vi "Assemble DC Rectifier Setting Changes for PLC.vi"(6 "Num Steps":i32, 7 "Rect Number":i32=1, 8 "error In":errorcluster, 10 "message queue in":T1, 11 "MulticolumnListbox in":refnum<vi>) -> (0 "Right Anode Mins":dbl, 1 "Left Anode Mins":dbl, 2 "Right AmpMin":dbl, 3 "Left AmpMin":dbl, 4 "error out":errorcluster)   [LabVIEW 2019]
uses:
  <vilib>/NI/AMC/Message Queue.ctl
  <vilib>/NI/AMC/Message.ctl
  <vilib>/NI/Tools/Keyed Array/KeyedArray.ctl
  <vilib>/NI/Current Value Table/Type Defs/Single Tag.ctl
  <vilib>/NI/Current Value Table/Type Defs/Data Types.ctl
  <vilib>/NI/AMC/Create Single Message.vi
  <vilib>/NI/AMC/Update Message Routing Info.vi
  <vilib>/NI/AMC/Send Message.vi
  <vilib>/NI/AMC/AMC.lvlib
  <vilib>/NI/Current Value Table/Current Value Table.lvlib
  <vilib>/NI/Tools/Keyed Array/Tools_KeyedArray.lvlib
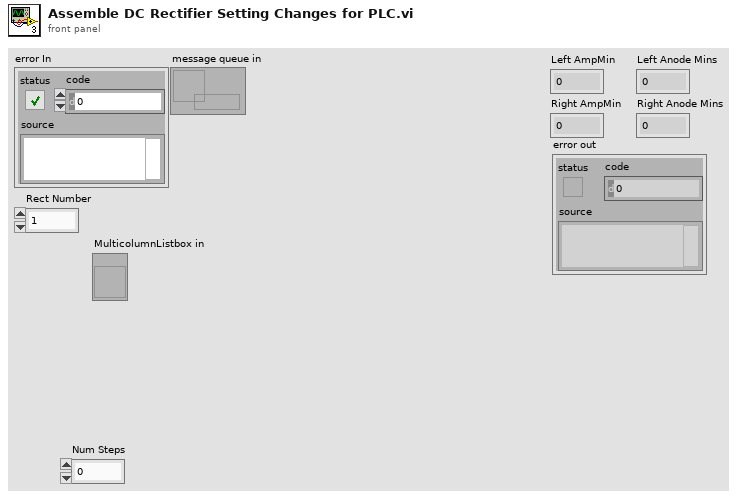
[diagram p1: front panel]
types:
  T1 = typedef "AMC.lvlib/Message Queue.ctl" = refnum<queue>
  T2 = typedef "Current Value Table.lvlib/Data Types.ctl" = enum16{"Double", "Single", "I64", "I32", "I16", "I8", "U64", "U32", "U16", "U8", "String", "Boolean", "Array of U8", "Array of U16", "Array of U32", "Array of U64", "Array of I64", "Array of I32", "Array of I16", "Array of I8", "Array of Double", "Array of Single", "Array of Boolean", "Array of String"}
  T3 = typedef "Current Value Table.lvlib/Single Tag.ctl" = cluster{"Data Type":T2, "Name":string, "Value":string, "Description":string}
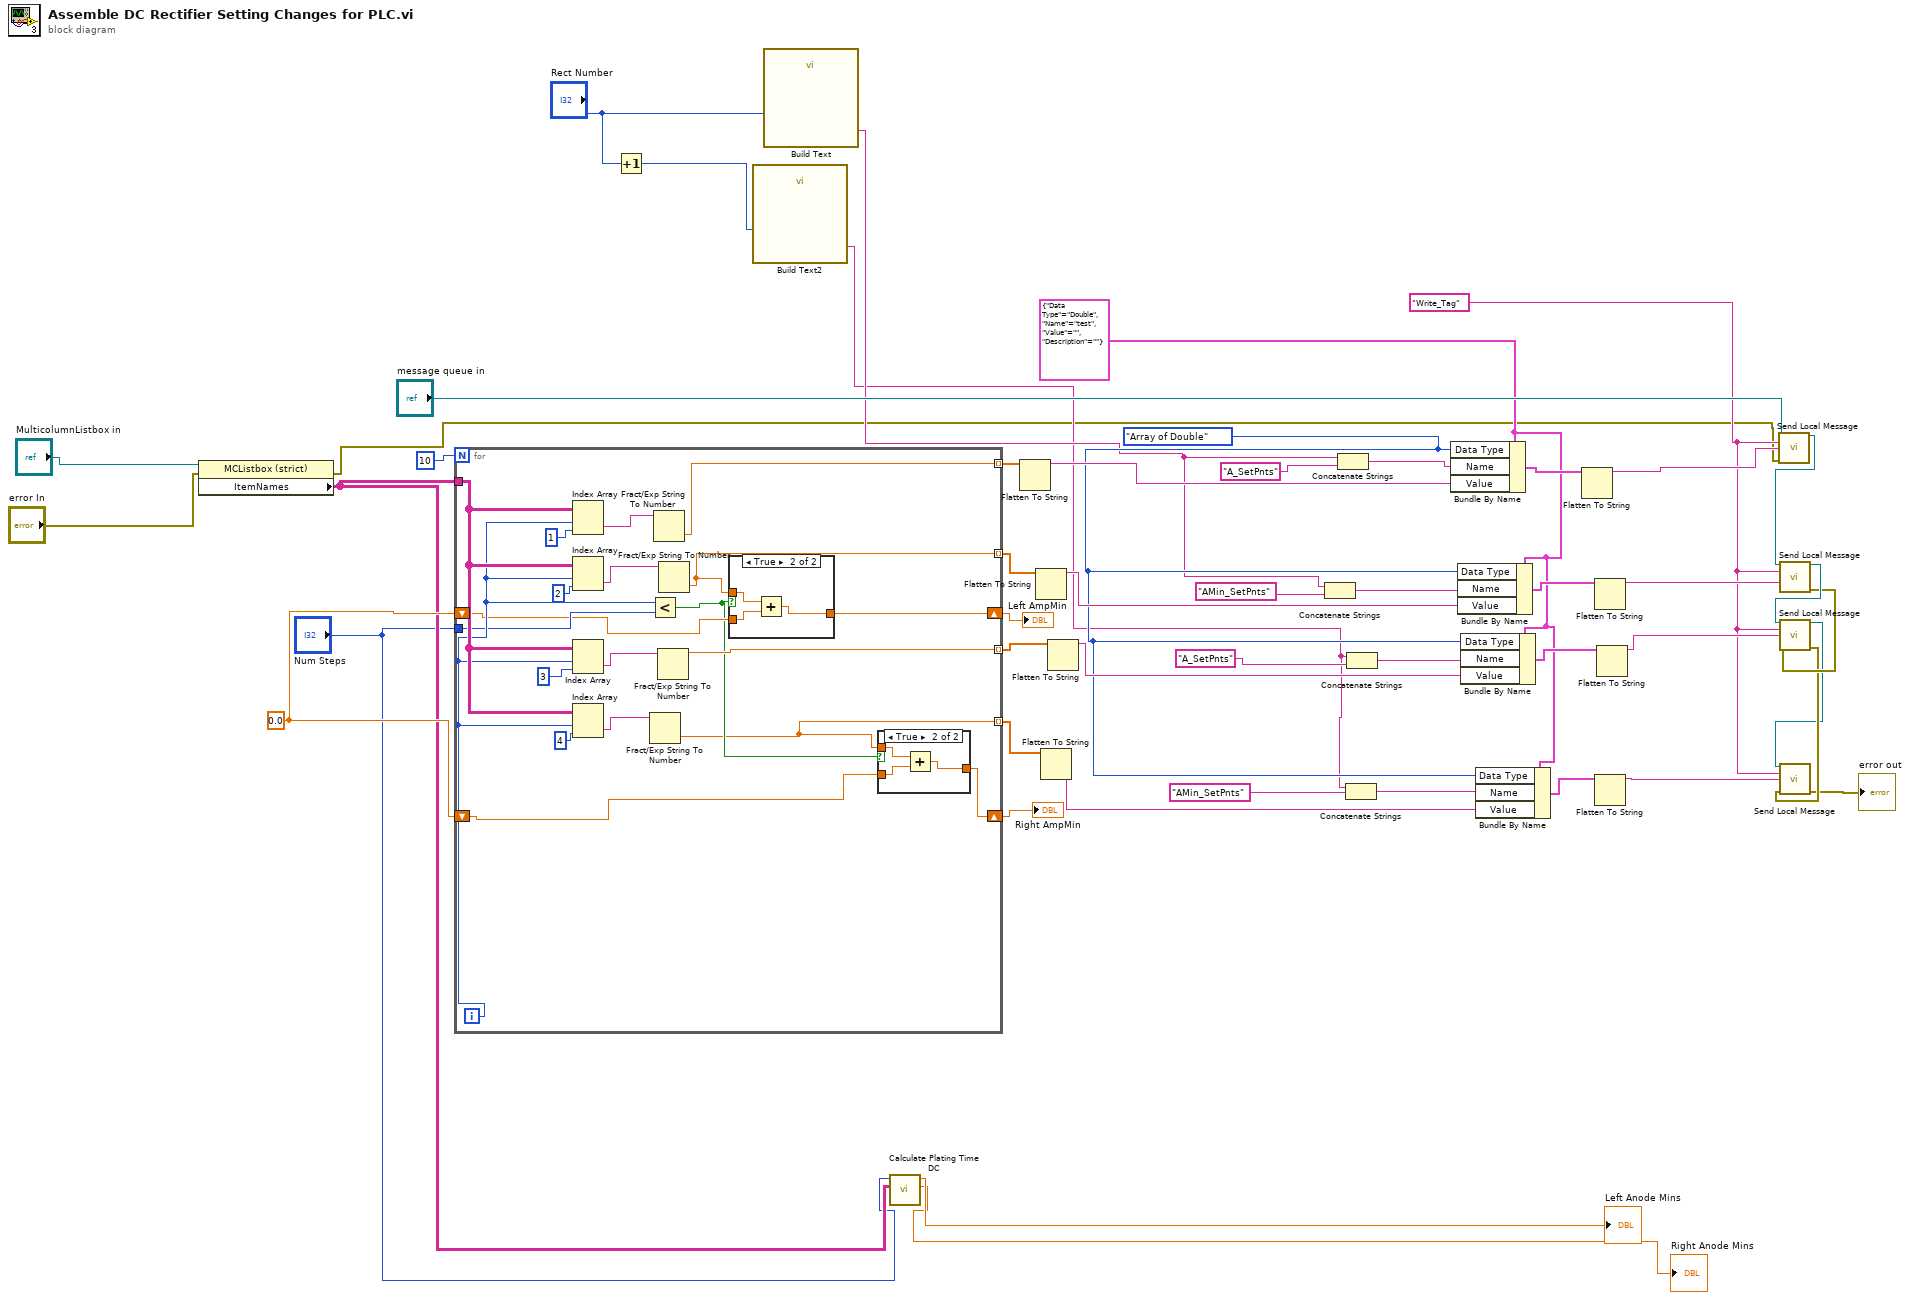
[diagram p0: block diagram]
diagram:
  w13 = 0.0
  w27 = Data_Types."Array of Double" ("Data Type")
  w28 = T3 {"Data Type"=enum."Double", "Name"="test", "Value"="", "Description"=""} ("Tag")
  w26 = "Write_Tag" ("message name")
  n1 = property class="MCListbox (strict)"(reference="MulticolumnListbox in", error in="error In") -> (error out=w12:errorcluster, "ItemNames"=w4:string[][])  [unwired: 1 out]
  n2 = for {
    N: 10 -> [_]
    tunnel: w4 -> [w64]
    tunnel: [w60] -> w46 mode=indexing
    tunnel: [w56] -> w41 mode=indexing
    tunnel: [w59] -> w37 mode=indexing
    tunnel: [w52] -> w32 mode=indexing
    tunnel: "Num Steps" -> [w57]
    shift-right: [w54] -> w10
    shift-left: w13 -> [w55]
    shift-right: [w50] -> w9
    shift-left: w13 -> [w51]
    i -> [w58]
    n3 = Index Array(array=w64, index (row)=w58, index (col)=1 ("disabled index (col)")) -> (element=w68:string)
    n4 = Index Array(array=w64, index (row)=w58, index (col)=2 ("disabled index (col)")) -> (element=w63:string)
    n5 = Index Array(array=w64, index (row)=w58, index (col)=3 ("disabled index (col)")) -> (element=w62:string)
    n6 = Index Array(array=w64, index (row)=w58, index (col)=4 ("disabled index (col)")) -> (element=w61:string)
    n7 = Less?(x=w58, y=w57) -> (x < y?=w53:bool)
    n8 = Fract/Exp String To Number(string=w61) -> (number=w52:dbl)  [unwired: 3 in, 1 out]
    n9 = Fract/Exp String To Number(string=w68) -> (number=w60:dbl)  [unwired: 3 in, 1 out]
    n10 = Fract/Exp String To Number(string=w62) -> (number=w59:dbl)  [unwired: 3 in, 1 out]
    n11 = Fract/Exp String To Number(string=w63) -> (number=w56:dbl)  [unwired: 3 in, 1 out]
    n12 = case shown="True" w53 {
      tunnel: w56 -> [_ w77]
      tunnel: w55 -> [w74 w76]
      tunnel: [w74 w75] -> w54
      frame False {
      }
      frame True {
        n13 = Add(x=w77, y=w76) -> (x+y=w75:dbl)
      }
    }
    n14 = case shown="True" w53 {
      tunnel: w52 -> [_ w73]
      tunnel: w51 -> [w70 w72]
      tunnel: [w70 w71] -> w50
      frame False {
      }
      frame True {
        n15 = Add(x=w73, y=w72) -> (x+y=w71:dbl)
      }
    }
  }
  "Left AmpMin" <- w10
  "Right AmpMin" <- w9
  n16 = Increment(x="Rect Number") -> (x+1=w24:i32)
  n17 = call "Build Text2"("Rect1"=w24) -> ("Result"=w15:string)  [unwired: 13 in, 1 out]
  n18 = call "Build Text"("Rect1"="Rect Number") -> ("Result"=w19:string)  [unwired: 13 in, 1 out]
  n19 = call "Calculate Plating Time DC.vi"("ItemNames"=w4, "Num Steps"="Num Steps") -> ("Right Anode Time"=→"Right Anode Mins":dbl, "Left Anode Time"=→"Left Anode Mins":dbl)  [unwired: 8 in]
  n20 = Flatten To String(anything=w46) -> (data string=w44:string)  [unwired: 3 in, 2 out]
  n21 = Flatten To String(anything=w41) -> (data string=w40:string)  [unwired: 3 in, 2 out]
  n22 = Flatten To String(anything=w32) -> (data string=w31:string)  [unwired: 3 in, 2 out]
  n23 = Flatten To String(anything=w37) -> (data string=w36:string)  [unwired: 3 in, 2 out]
  n24 = Concatenate Strings(w19, "AMin_SetPnts" ("Name")) -> (w21:string)
  n25 = Concatenate Strings(w19, "A_SetPnts" ("Name")) -> (w23:string)
  n26 = Concatenate Strings(w15, "AMin_SetPnts" ("Name")) -> (w16:string)
  n27 = Concatenate Strings(w15, "A_SetPnts" ("Name")) -> (w17:string)
  n28 = Bundle By Name(cluster=w28, "Data Type"=w27, "Name"=w23, "Value"=w44) -> (w43:T3)
  n29 = Bundle By Name(cluster=w28, "Data Type"=w27, "Name"=w21, "Value"=w40) -> (w39:T3)
  n30 = Bundle By Name(cluster=w28, "Data Type"=w27, "Name"=w17, "Value"=w36) -> (w35:T3)
  n31 = Bundle By Name(cluster=w28, "Data Type"=w27, "Name"=w16, "Value"=w31) -> (w30:T3)
  n32 = Flatten To String(anything=w43) -> (data string=w42:string)  [unwired: 3 in, 2 out]
  n33 = Flatten To String(anything=w39) -> (data string=w38:string)  [unwired: 3 in, 2 out]
  n34 = Flatten To String(anything=w30) -> (data string=w29:string)  [unwired: 3 in, 2 out]
  n35 = Flatten To String(anything=w35) -> (data string=w33:string)  [unwired: 3 in, 2 out]
  n36 = call <vilib>:"Send Local Message.vi"("message queue in"="message queue in", "message name"=w26, "message value"=w42, "error in"=w12) -> ("message queue out"=w8:T1)  [unwired: 9 in, 2 out]
  n37 = call <vilib>:"Send Local Message.vi"("message queue in"=w8, "message name"=w26, "message value"=w38) -> ("message queue out"=w34:T1, "error out"=w11:errorcluster)  [unwired: 10 in, 1 out]
  n38 = call <vilib>:"Send Local Message.vi"("message queue in"=w34, "message name"=w26, "message value"=w33, "error in"=w11) -> ("message queue out"=w6:T1, "error out"=w7:errorcluster)  [unwired: 9 in, 1 out]
  n39 = call <vilib>:"Send Local Message.vi"("message queue in"=w6, "message name"=w26, "message value"=w29, "error in"=w7) -> ("error out"=→"error out":errorcluster)  [unwired: 9 in, 2 out]
